vi "23384_Davis_Poku_Amankwa_Amankwa.DavisPoku.MNE1201.4.DIY_348257_1982665141.vi"() -> ()   [LabVIEW 2018]
uses:
  <vilib>/imath/engines/lvmath2/RunTimeEngine/Managers/WorkSpace/UID Generator.vi
  <vilib>/imath/engines/lvmath2/RunTimeEngine/RunTimeType/NIMS_RunTimeType_From StrictType (excl LVString).vi
  <instcachedir>/0/NIMS_RunTimeType_From StrictType (excl LVString)_E7E34A65C99947108168652BAD14964D.lvgen/NIMS_RunTimeType_From StrictType (excl LVString)_E7E34A65C99947108168652BAD14964D_000.vi
  <vilib>/imath/engines/lvmath2/RunTimeEngine/LocalVariableDefStatement/MC_LocalVariableDefStatement_Display.vi
  <vilib>/imath/engines/lvmath2/RunTimeEngine/RangeToken/NIMS_Range.vi
  <instcachedir>/0/NIMS_Range_846134F467D14A349F7C6CCEF459CDB2.lvgen/NIMS_Range_846134F467D14A349F7C6CCEF459CDB2_000.vi
  <vilib>/imathl/engines/lvmath/Functions/Error Handling/Create Error.vi
  <vilib>/imath/engines/lvmath2/RunTimeEngine/ArithmeticOperatorToken/NIMS_ArithmeticOperator_times.vi
  <instcachedir>/0/NIMS_ArithmeticOperator_times_D7E4A7A4AD2C4409A0CE309D2741A5B4.lvgen/NIMS_ArithmeticOperator_times_D7E4A7A4AD2C4409A0CE309D2741A5B4_000.vi
  <vilib>/imath/engines/lvmath2/RunTimeEngine/Managers/SymbolTable/Clear UID.vi
  <vilib>/imath/engines/lvmath2/RunTimeEngine/NodeEndStatement/NIMS_NodeEndStatement_Output.vi
  <instcachedir>/0/NIMS_NodeEndStatement_Output_53EC0D466D134D7ABD903AC30B43404B.lvgen/NIMS_NodeEndStatement_Output_53EC0D466D134D7ABD903AC30B43404B_005.vi
  <vilib>/imath/engines/lvmath2/RunTimeEngine/ErrorHandling/NIMS_Finalize Error.vi
  <vilib>/imath/engines/lvmath2/RunTimeEngine/Managers/SymbolTable/NIMS_WorkSpace.lvlib
panel:
  out "AM WAVE":cluster{"Time":dbl[], "Disp;lacement":dbl[]}
  in  "AM PARAMETERS":T1
  in  "Digitizing Parameters":T2
  out "XY Graph":cluster{"t":dbl[], "x":dbl[]}(graph)
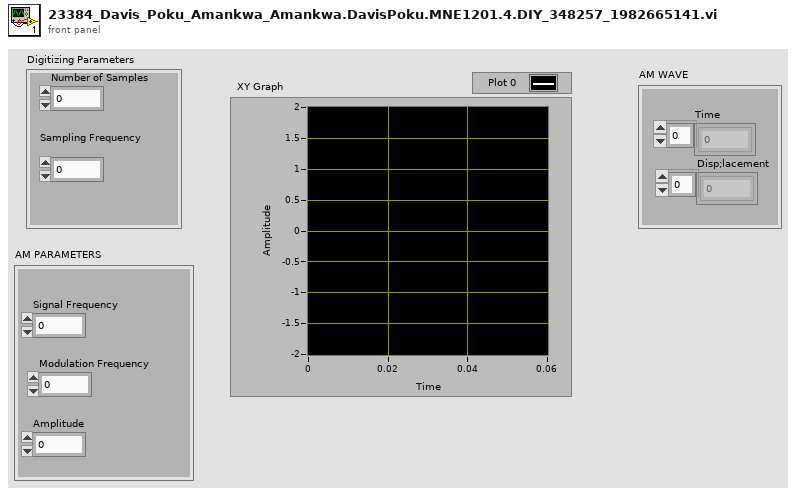
[diagram p1: front panel]
types:
  T1 = cluster{"Signal Frequency":dbl, "Modulation Frequency":dbl, "Amplitude":dbl}
  T2 = cluster{"Number of Samples":dbl, "Sampling Frequency":dbl}
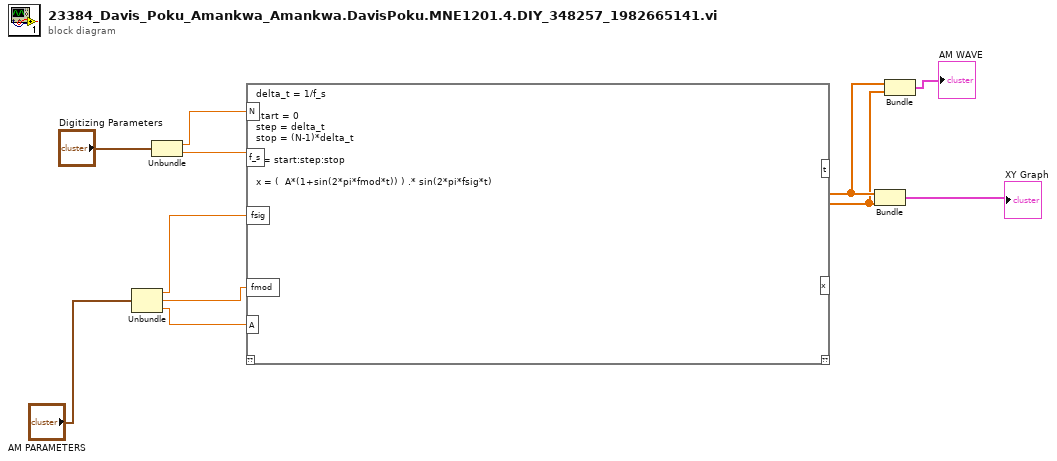
[diagram p0: block diagram]
diagram:
  n1 = Unbundle("AM PARAMETERS") -> ("Signal Frequency"=w6:dbl, "Modulation Frequency"=w5:dbl, "Amplitude"=w4:dbl)
  n2 = Unbundle("Digitizing Parameters") -> ("Number of Samples"=w2:dbl, "Sampling Frequency"=w1:dbl)
  n3 = mathscript code="delta_t = 1/f_s\n\nstart = 0 \nstep = delta_t\nstop = (N-1)*delta_t\n\nt = start:step:stop\n\nx = (  A*(1+sin(2*pi*fmod*t)) ) .* sin(2*pi*fsig*t)"("N"=w2, "f_s"=w1, "fsig"=w6, "fmod"=w5, "A"=w4) -> ("t"=w10:dbl[], "x"=w9:dbl[])  [unwired: 1 in, 1 out]
  n4 = Bundle("t"=w10, "x"=w9) -> (→"XY Graph":cluster{"t":dbl[], "x":dbl[]})  [unwired: 1 in]
  n5 = Bundle("t"=w10, "x"=w9) -> (→"AM WAVE":cluster{"t":dbl[], "x":dbl[]})  [unwired: 1 in]
